vi "LookupTableBuild.vi"(11 "sub-system cfgs":T2[](array[typedef])) -> (3 "Lookup Table":T1(array[cluster]))   [LabVIEW 2019]
uses:
  VXMCfg/sub-syst.n.ctl
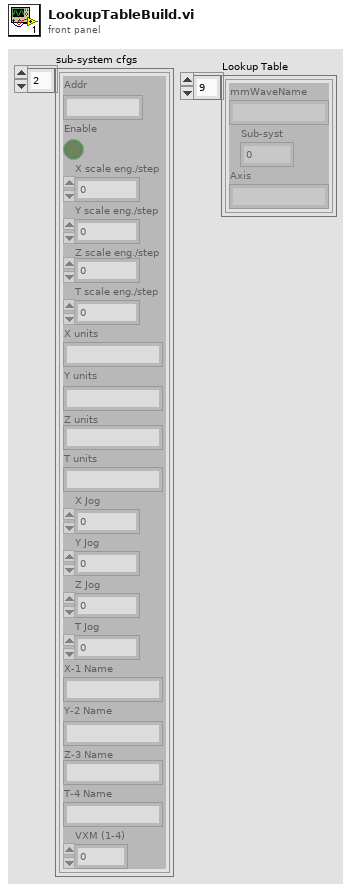
[diagram p1: front panel]
types:
  T1 = cluster{"mmWaveName":string, "Sub-syst":i32, "Axis":string}[]
  T2 = typedef "sub-syst.n.ctl" = cluster{"Addr":string, "Enable":bool, "X scale eng./step":dbl, "Y scale eng./step":dbl, "Z scale eng./step":dbl, "T scale eng./step":dbl, "X units":string, "Y units":string, "Z units":string, "T units":string, "X Jog":dbl, "Y Jog":dbl, "Z Jog":dbl, "T Jog":dbl, "X-1 Name":string, "Y-2 Name":string, "Z-3 Name":string, "T-4 Name":string, "VXM (1-4)":i32}
  T3 = cluster{"mmWaveName":string, "Sub-syst":i32, "Axis":string}
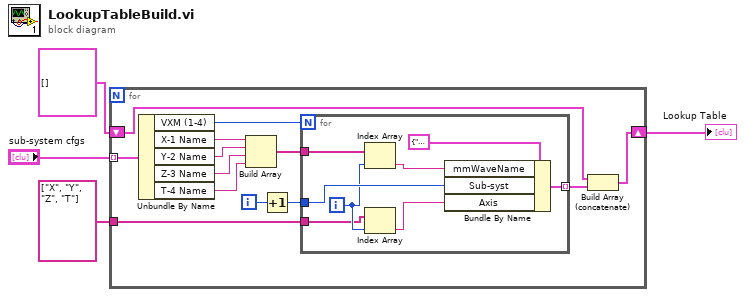
[diagram p0: block diagram]
diagram:
  n1 = for {
    tunnel: "sub-system cfgs" -> [w17] mode=indexing
    tunnel: string[] ["X", "Y", "Z", "T"] -> [w8]
    shift-right: [w5] -> w1
    shift-left: T1 [] -> [w6]
    i -> [w15]
    n2 = Unbundle By Name(w17) -> ("VXM (1-4)"=w14:i32, "X-1 Name"=w13:string, "Y-2 Name"=w12:string, "Z-3 Name"=w11:string, "T-4 Name"=w10:string)
    n3 = Build Array(w13, w12, w11, w10) -> (w9:string[])
    n4 = Increment(x=w15) -> (x+1=w16:i32)
    n5 = for {
      N: w14 -> [_]
      tunnel: w16 -> [w25]
      tunnel: w9 -> [w24]
      tunnel: w8 -> [w21]
      tunnel: [w19] -> w7 mode=indexing
      i -> [w22]
      n6 = Index Array(array=w24, index=w22) -> (element=w23:string)
      n7 = Index Array(array=w21, index=w22) -> (element=w20:string)
      n8 = Bundle By Name(cluster=T3 {"mmWaveName"="", "Sub-syst"=0, "Axis"=""} ("output cluster"), "mmWaveName"=w23, "Sub-syst"=w25, "Axis"=w20) -> (w19:T3)
    }
    n9 = Build Array (concatenate)(w6, w7) -> (w5:T1)
  }
  "Lookup Table" <- w1
